vi "smart_temp_humid.vi"() -> ()   [LabVIEW 2021]
uses:
  <vilib>/LabVIEW Interface for Arduino/Type Defs/Pin Mode.ctl
  <vilib>/Utility/file.llb/Read Delimited Spreadsheet (string).vi
  <vilib>/Utility/file.llb/Write Delimited Spreadsheet (string).vi
  <vilib>/LabVIEW Interface for Arduino/LabVIEW Interface for Arduino.lvlib
  projet_ds/LIFA DHT11 LV9/DHT11.lvlib
panel:
  out "error out":errorcluster
  out "first row":string[](array[string])
  out "état de fonctionnement":string
  out "?":u8
  out "?":u8
  in  "IOT_DATA":bool
  out "Ventilateur":bool
  out "Climatiseur":bool
  in  "Initialisation":bool
  in  "Climatiseur":bool
  in  "ventillateur":bool
  out "Capteur DHT11":bool
  out "Humidite":dbl(knob) scale=0.0..255.0
  in  "VISA resource":refnum<visa-resource-name>
  out "temperature":dbl(slide) scale=0.0..255.0
  in  "?":bool
  in  "?":bool
  in  "Send_info":bool
  in  "Mail :":string="dhiadridi06@gmail.com"
  out "XY Plot Matrix":cluster{"all rows":dbl[], "all rows":dbl[]}(graph)
  out "plot":errorcluster
  out "errreure humidité":errorcluster
  out "erreur temperature":errorcluster
  out "error out 2":errorcluster
  # "dhaouidridi20434792@gmail.com"
  # "Gestion intelligente : temperature et     \n                                humidité"
  # "Visualisation"
  # "AUTO_MANU"
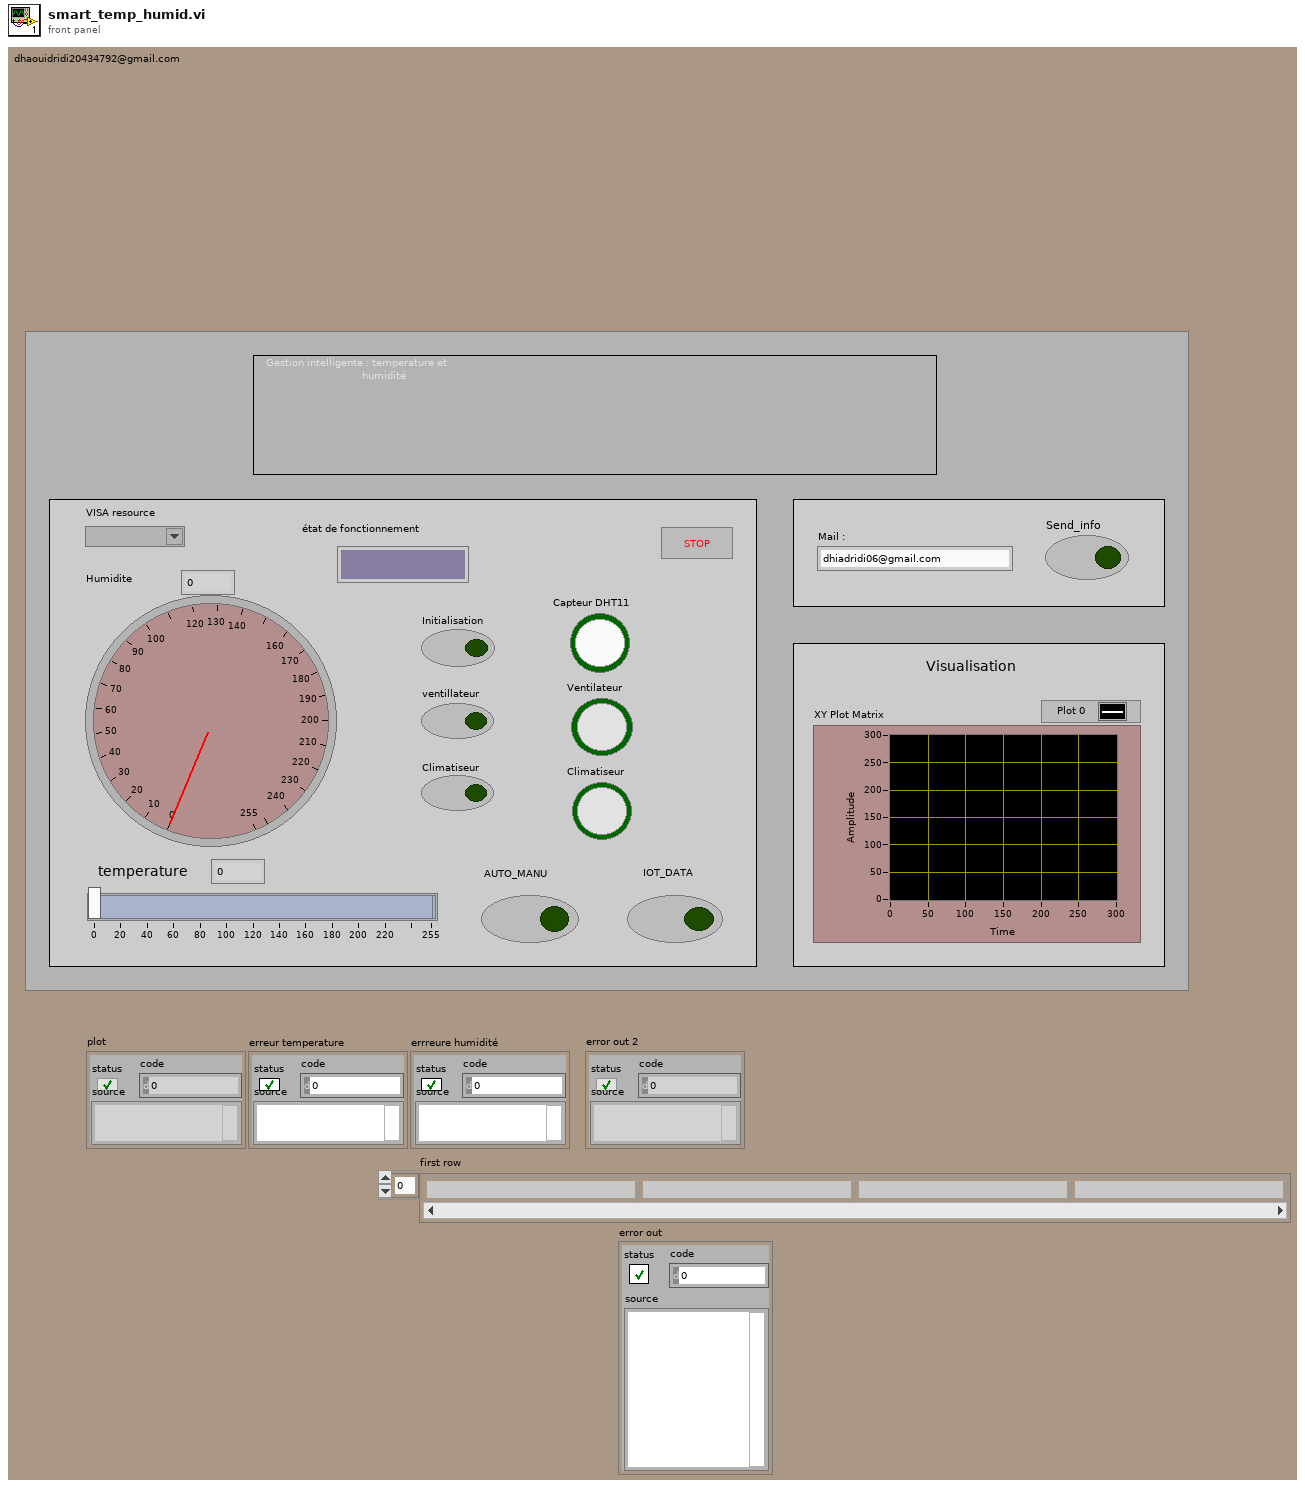
[diagram p1: front panel]
types:
  T1 = typedef "LabVIEW Interface for Arduino.lvlib/Arduino Resource.ctl" = cluster{"VISA resource":refnum<visa-resource-name>, "Board Type":T2, "Connection Type":enum8{"USB / Serial"}, "Bytes Per Packet (15)":u8}
  T2 = typedef "LabVIEW Interface for Arduino.lvlib/Board Type.ctl" = enum16{"Uno", "Dimuelanove w/Atmega 328", "Mega 2560"}
  T3 = typedef "LabVIEW Interface for Arduino.lvlib/Pin Mode.ctl" = enum8{"Input", "Output"}
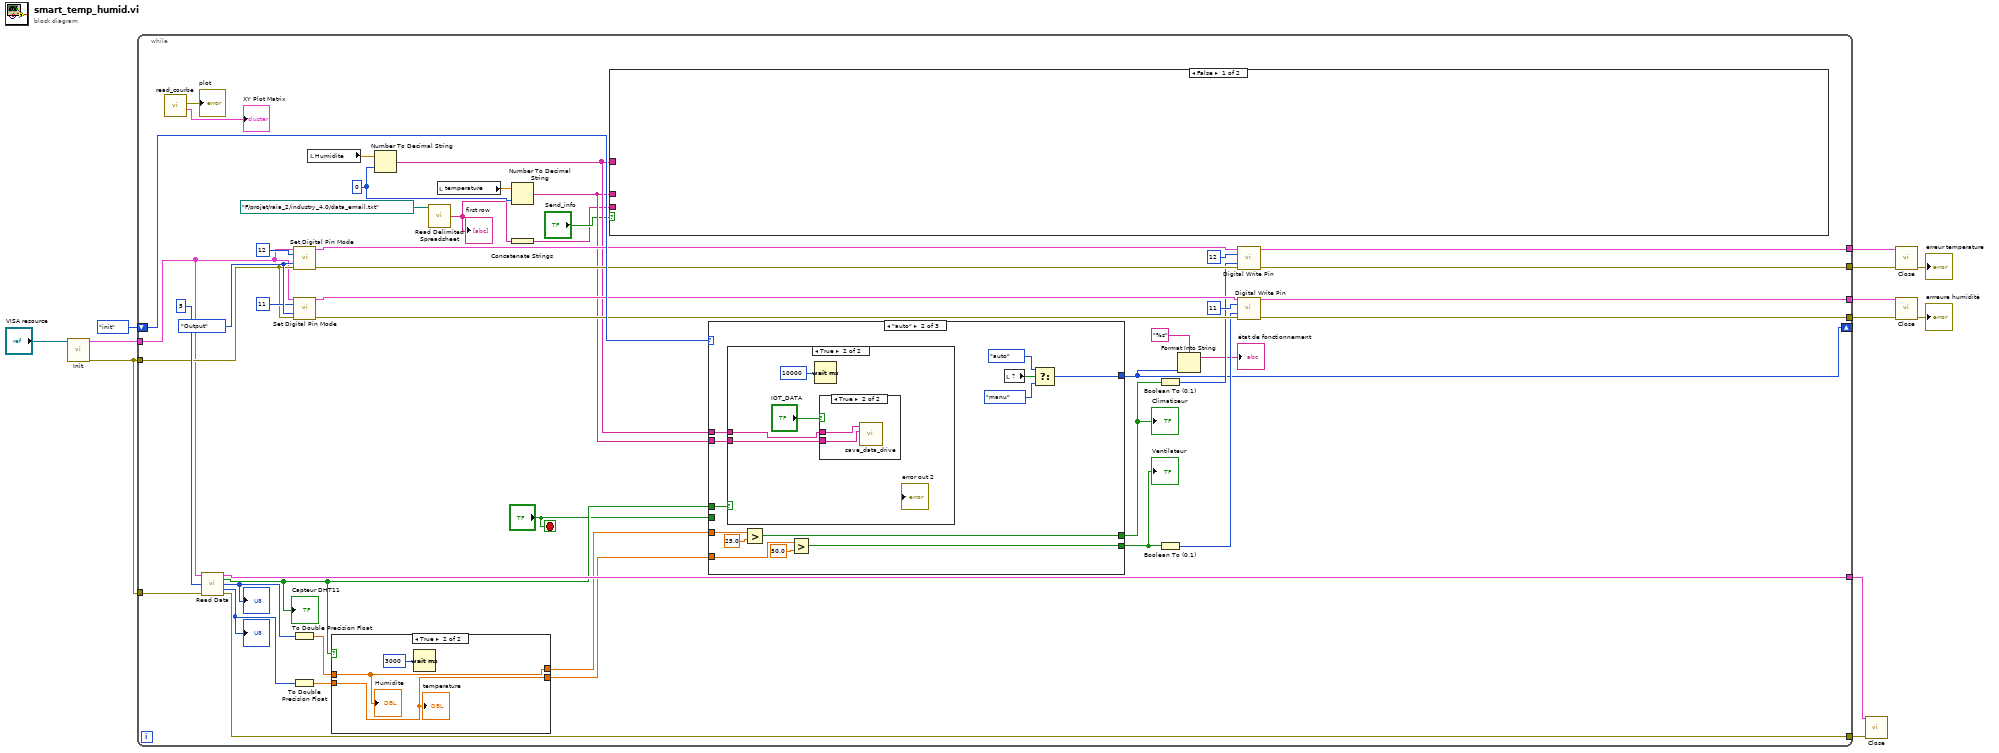
[diagram p0: block diagram]
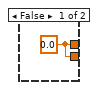
[diagram p2: hidden frame]
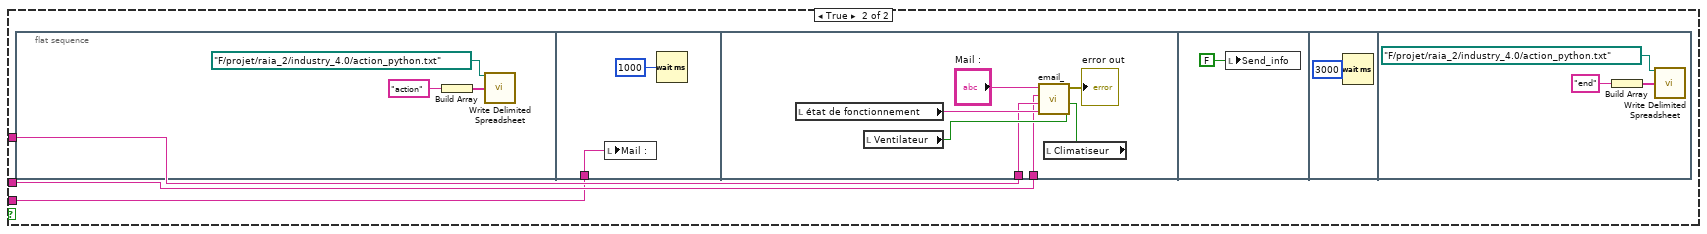
[diagram p3: hidden frame]
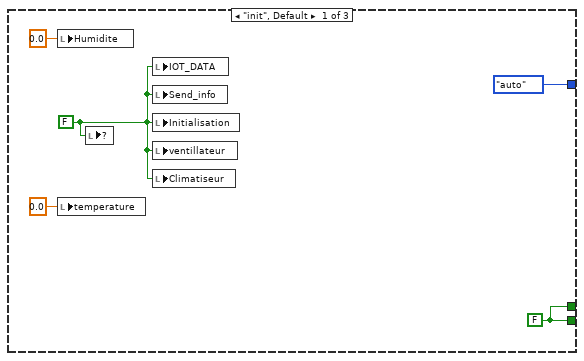
[diagram p4: hidden frame]
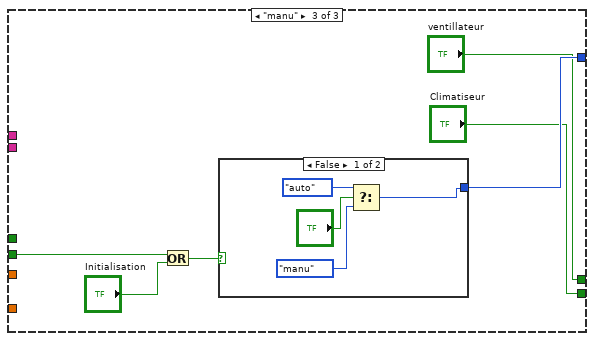
[diagram p7: hidden frame]
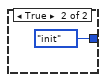
[diagram p8: hidden frame]
diagram:
  n1 = call <vilib>:"Init.vi"("VISA resource"="VISA resource") -> ("Arduino Resource"=w10:T1, "error out"=w3:errorcluster)  [unwired: 17 in]
  n2 = while {
    shift-right: [w23] -> _
    shift-left: enum16{"init", "auto", "manu"}."init" -> [w58]
    tunnel: w10 -> [w40]
    tunnel: w3 -> [w39]
    tunnel: [w53] -> w7
    tunnel: [w52] -> w6
    tunnel: [w51] -> w5
    tunnel: [w50] -> w4
    tunnel: w3 -> [w46]
    tunnel: [w38] -> w2
    tunnel: [w37] -> w1
    stop <- "?" stop-if-true
    w28 = i16 0 ("width (-)")
    w48 = Pin_Mode."Output" ("Pin Mode (Input)")
    n3 = call "read_courbe.vi"() -> ("XY Plot Matrix"=→"XY Plot Matrix":cluster{"all rows":dbl[], "all rows":dbl[]}, "error out"=→"plot":errorcluster)  [unwired: 10 in]
    n4 = call "Read Data.vi"("Arduino Resource"=w40, "Pin"=u8 5 ("Digital I/O Pin (0)"), "error in (no error)"=w39) -> ("Arduino Resource"=w38:T1, "Successful?"=w34:bool, "Relative Humidity"=w56:u8, "Temperature (°C)"=w41:u8, "error out"=w37:errorcluster)  [unwired: 8 in]
    "Capteur DHT11" <- w34
    "?" <- w56
    "?" <- w41
    n5 = call <vilib>:"Set Digital Pin Mode.vi"("Arduino Resource"=w40, "Digital I/O Pin"=u8 12, "Pin Mode (Input)"=w48, "error in"=w46) -> ("Arduino Resource"=w43:T1, "error out"=w42:errorcluster)  [unwired: 10 in]
    n6 = call <vilib>:"Set Digital Pin Mode.vi"("Arduino Resource"=w40, "Digital I/O Pin"=u8 11, "Pin Mode (Input)"=w48, "error in"=w46) -> ("Arduino Resource"=w45:T1, "error out"=w44:errorcluster)  [unwired: 10 in]
    n7 = To Double Precision Float(number=w56) -> (double precision float=w17:dbl)
    n8 = To Double Precision Float(number=w41) -> (double precision float=w16:dbl)
    n9 = local read "Humidite"() -> (w19:dbl)
    n10 = case shown="True" w34 {
      tunnel: w17 -> [_ w62]
      tunnel: w16 -> [_ w61]
      tunnel: [w59 w62] -> w15
      tunnel: [w59 w61] -> w14
      frame False {
        w59 = 0.0
      }
      frame True {
        n11 = Wait (ms)(milliseconds to wait=u32 3000) -> ()  [unwired: 1 out]
        "Humidite" <- w62
        "temperature" <- w61
      }
    }
    n12 = Number To Decimal String(number=w19, width (-)=w28) -> (decimal integer string=w27:string)
    n13 = call-poly <vilib>:"Read Delimited Spreadsheet.vi"("file path (dialog if empty)"=path "F:/projet/raia_2/industry_4.0/data_email.txt") -> ("first row"=w20:string[])  [unwired: 9 in, 5 out]
    "first row" <- w20
    n14 = local read "temperature"() -> (w18:dbl)
    n15 = Number To Decimal String(number=w18, width (-)=w28) -> (decimal integer string=w26:string)
    n16 = Concatenate Strings(w20) -> (w13:string)
    n17 = case shown="False" "Send_info" {
      tunnel: w26 -> [_ w64]
      tunnel: w27 -> [_ w65]
      tunnel: w13 -> [_ w63]
      frame False {
      }
      frame True {
        n18 = flat-sequence {
          tunnel: w63 -> [w69]
          tunnel: w65 -> [w74]
          tunnel: w64 -> [w73]
          frame #0 {
            n19 = Build Array("action" ("String")) -> (w66:string[])
            n20 = call-poly <vilib>:"Write Delimited Spreadsheet.vi"("file path (dialog if empty)"=path "F:/projet/raia_2/industry_4.0/action_python.txt", "1D data"=w66) -> ()  [unwired: 12 in, 2 out]
          }
          frame #1 {
            n21 = local write "Mail :"(w69) -> ()
            n22 = Wait (ms)(milliseconds to wait=u32 1000) -> ()  [unwired: 1 out]
          }
          frame #2 {
            n23 = local read "état de fonctionnement"() -> (w77:string)
            n24 = local read "Ventilateur"() -> (w76:bool)
            n25 = local read "Climatiseur"() -> (w75:bool)
            n26 = call "email_.vi"("vent"=w76, "clim"=w75, "mode"=w77, "humid"=w74, "temp"=w73, "to"="Mail :") -> ("error out"=→"error out":errorcluster)  [unwired: 5 in]
          }
          frame #3 {
            n27 = local write "Send_info"(FALSE ("Send_info")) -> ()
          }
          frame #4 {
            n28 = Wait (ms)(milliseconds to wait=u32 3000) -> ()  [unwired: 1 out]
          }
          frame #5 {
            n29 = Build Array("end" ("String")) -> (w80:string[])
            n30 = call-poly <vilib>:"Write Delimited Spreadsheet.vi"("file path (dialog if empty)"=path "F:/projet/raia_2/industry_4.0/action_python.txt", "1D data"=w80) -> ()  [unwired: 12 in, 2 out]
          }
        }
      }
    }
    n31 = case shown="\"auto\"" w58 {
      tunnel: [enum16{"init", "auto", "manu"}."auto" w100 w112] -> w23
      tunnel: w34 -> [_ w90 _]
      tunnel: "?" -> [_ _ w109]
      tunnel: [w84 w94 "Climatiseur"] -> w30
      tunnel: [w84 w93 "ventillateur"] -> w29
      tunnel: w27 -> [_ w92 _]
      tunnel: w26 -> [_ w91 _]
      tunnel: w15 -> [_ w89 _]
      tunnel: w14 -> [_ w88 _]
      frame "init", Default {
        w84 = FALSE ("clim")
        w83 = FALSE ("ventillateur")
        n32 = local write "Humidite"(0.0) -> ()
        n33 = local write "temperature"(0.0) -> ()
        n34 = local write item#1(w83) -> ()
        n35 = local write "IOT_DATA"(w83) -> ()
        n36 = local write "Send_info"(w83) -> ()
        n37 = local write "Initialisation"(w83) -> ()
        n38 = local write "ventillateur"(w83) -> ()
        n39 = local write "Climatiseur"(w83) -> ()
      }
      frame "auto" {
        n40 = case shown="True" w90 {
          tunnel: w92 -> [_ w101]
          tunnel: w91 -> [_ w102]
          frame False {
          }
          frame True {
            n41 = Wait (ms)(milliseconds to wait=u32 10000) -> ()  [unwired: 1 out]
            n42 = case shown="True" "IOT_DATA" {
              tunnel: w102 -> [_ w106]
              tunnel: w101 -> [_ w105]
              frame False {
              }
              frame True {
                n43 = call "save_data_drive.vi"("element 2"=w106, "element"=w105) -> ()  [unwired: 10 in]
              }
            }
          }
        }
        n44 = Greater?(x=w89, y=25.0) -> (0:w93:bool)
        n45 = Greater?(x=w88, y=50.0) -> (0:w94:bool)
        n46 = local read item#1() -> (w97:bool)
        n47 = Select(t=enum16{"init", "auto", "manu"}."auto", s=w97, f=enum16{"init", "auto", "manu"}."manu") -> (s? t:f=w100:enum16{"init", "auto", "manu"})
      }
      frame "manu" {
        n48 = Or(x=w109, y="Initialisation") -> (x .or. y?=w110:bool)
        n49 = case shown="False" w110 {
          tunnel: [w114 enum16{"init", "auto", "manu"}."init"] -> w112
          frame False {
            n50 = Select(t=enum16{"init", "auto", "manu"}."auto", s="?", f=enum16{"init", "auto", "manu"}."manu") -> (s? t:f=w114:enum16{"init", "auto", "manu"})
          }
          frame True {
          }
        }
      }
    }
    "Ventilateur" <- w30
    "Climatiseur" <- w29
    n51 = Boolean To (0,1)(Boolean=w29) -> (0, 1=w31:i16)
    n52 = Boolean To (0,1)(Boolean=w30) -> (0, 1=w32:i16)
    n53 = Format Into String(format string="%s", w23) -> (resulting string=→"état de fonctionnement":string)  [unwired: 2 in, 1 out]
    n54 = call <vilib>:"Digital Write Pin.vi"("Arduino Resource"=w43, "Digital I/O Pin (0)"=u8 12, "Value (0)"=w31, "error in"=w42) -> ("Arduino Resource"=w51:T1, "error out"=w50:errorcluster)  [unwired: 10 in]
    n55 = call <vilib>:"Digital Write Pin.vi"("Arduino Resource"=w45, "Digital I/O Pin (0)"=u8 11, "Value (0)"=w32, "error in"=w44) -> ("Arduino Resource"=w53:T1, "error out"=w52:errorcluster)  [unwired: 10 in]
  }
  n56 = call <vilib>:"Close.vi"("Arduino Resource"=w2, "error in"=w1) -> ()  [unwired: 13 in, 1 out]
  n57 = call <vilib>:"Close.vi"("Arduino Resource"=w5, "error in"=w4) -> ("error out"=→"erreur temperature":errorcluster)  [unwired: 13 in]
  n58 = call <vilib>:"Close.vi"("Arduino Resource"=w7, "error in"=w6) -> ("error out"=→"errreure humidité":errorcluster)  [unwired: 13 in]
